vi "Add Startup VI.vi"(8 "error in (no error)":errorcluster, 10 "ProjectItem Refnum":refnum<vi>, 11 "EXE in":refnum<class "NI_AB_API_EXE.lvclass">) -> (0 "error out":errorcluster, 3 "EXE out":refnum<class "NI_AB_API_EXE.lvclass">)   [LabVIEW 2020, in "NI_AB_API_EXE.lvclass"]
uses:
  <vilib>/AppBuilder/AB_API/EXE/NI_AB_API_EXE.lvclass
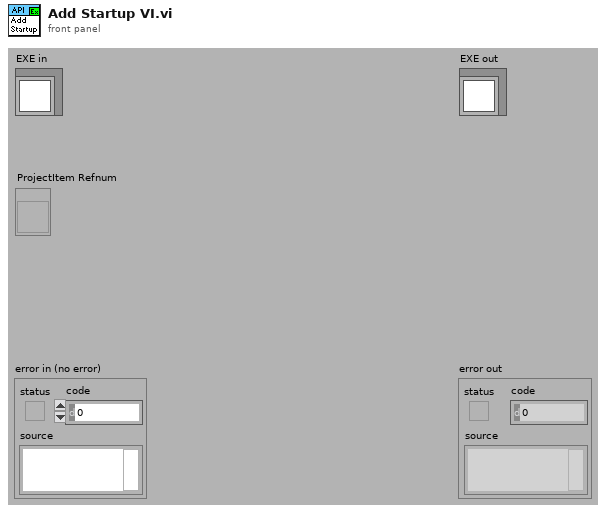
[diagram p1: front panel]
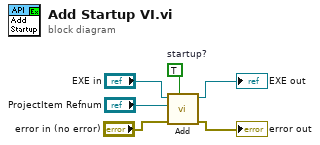
[diagram p0: block diagram]
diagram:
  w4 = TRUE  # startup?
  n1 = call <vilib>:"Add.vi"("startup?"=w4, "error in (no error)"="error in (no error)", "ProjectItem Refnum"="ProjectItem Refnum", "EXE in"="EXE in") -> ("error out"=→"error out":errorcluster, "EXE out"=→"EXE out":refnum<class "NI_AB_API_EXE.lvclass">)  [unwired: 6 in]
